vi "Test Parsing Simple Example Whlie Loop Some Operations 2.vi"() -> ()   [LabVIEW 2014]
panel:
  out "Transcripted code":string
  out "SubVI C calls":string[](array[string])
  out "error out 2":errorcluster
  out "WhileLoop C calls":string[](array[string])
  out "element translation order":string[](array[string])
  in  "vi path":path=path "C:/Users/lubo/Documents/LabView/LabVIEW-Universal-Transcriptor/Test/Examples For Parsing/Example While Loop Some Operations 2.vi"
  # "Everything is for noqw stored inside string list, so it means that all callected WhileLoops, SubVIs transcripted C code are store separately and after parsing there is generating them to output, but they are interleaved instead recursive nested, so this is what needs to repair next."
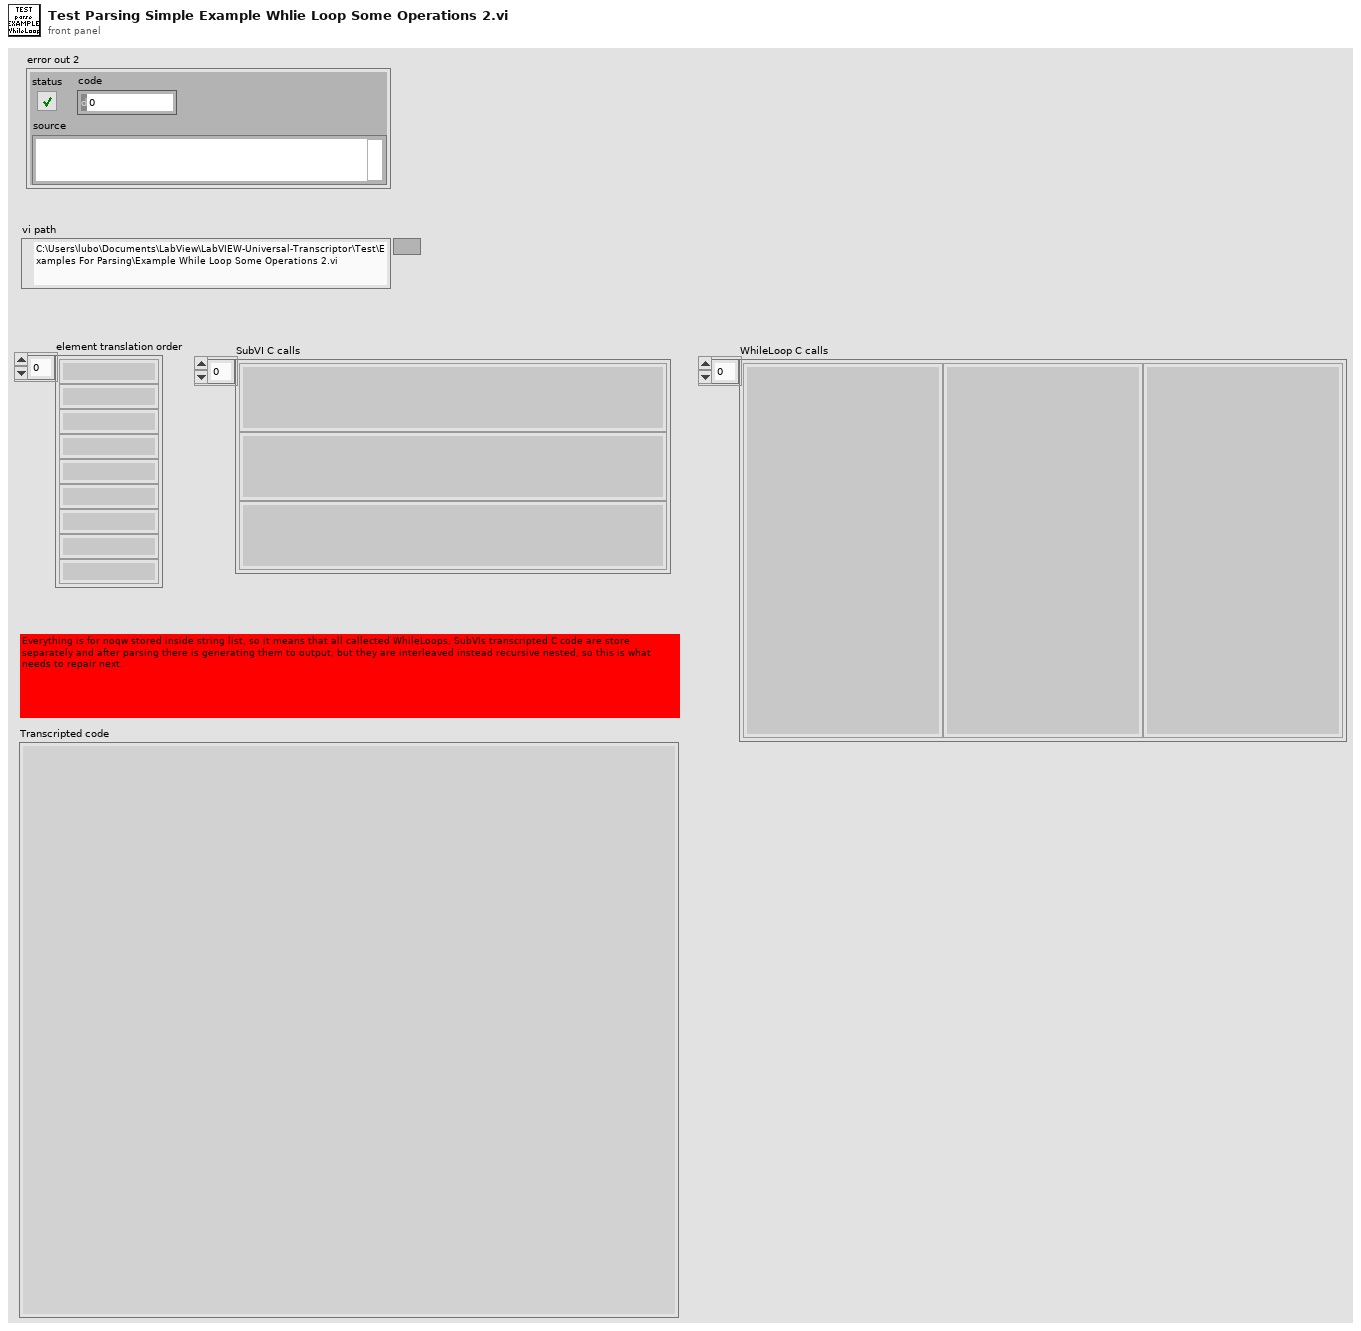
[diagram p1: front panel]
types:
  T1 = cluster{"terminals datatypes":string[][], "terminal\nconnected?":bool[], "terminal captions":string[], "term. count":i32, "terminal\nIsSource?":bool[], "SubVI name":string, "connected\nwires refs.":refnum<vi>[], "coerced\ndot?":bool[], "terminals[]":refnum<vi>[]}
  T2 = cluster{"terminals datatypes":string[][], "terminal\nconnected?":bool[], "terminal captions":string[], "term. count":i32, "terminal\nIsSource?":bool[], "SubVI name":string, "connected\nwires refs.":refnum<vi>[], "coerced dot?":bool[], "terminals[]":refnum<vi>[]}
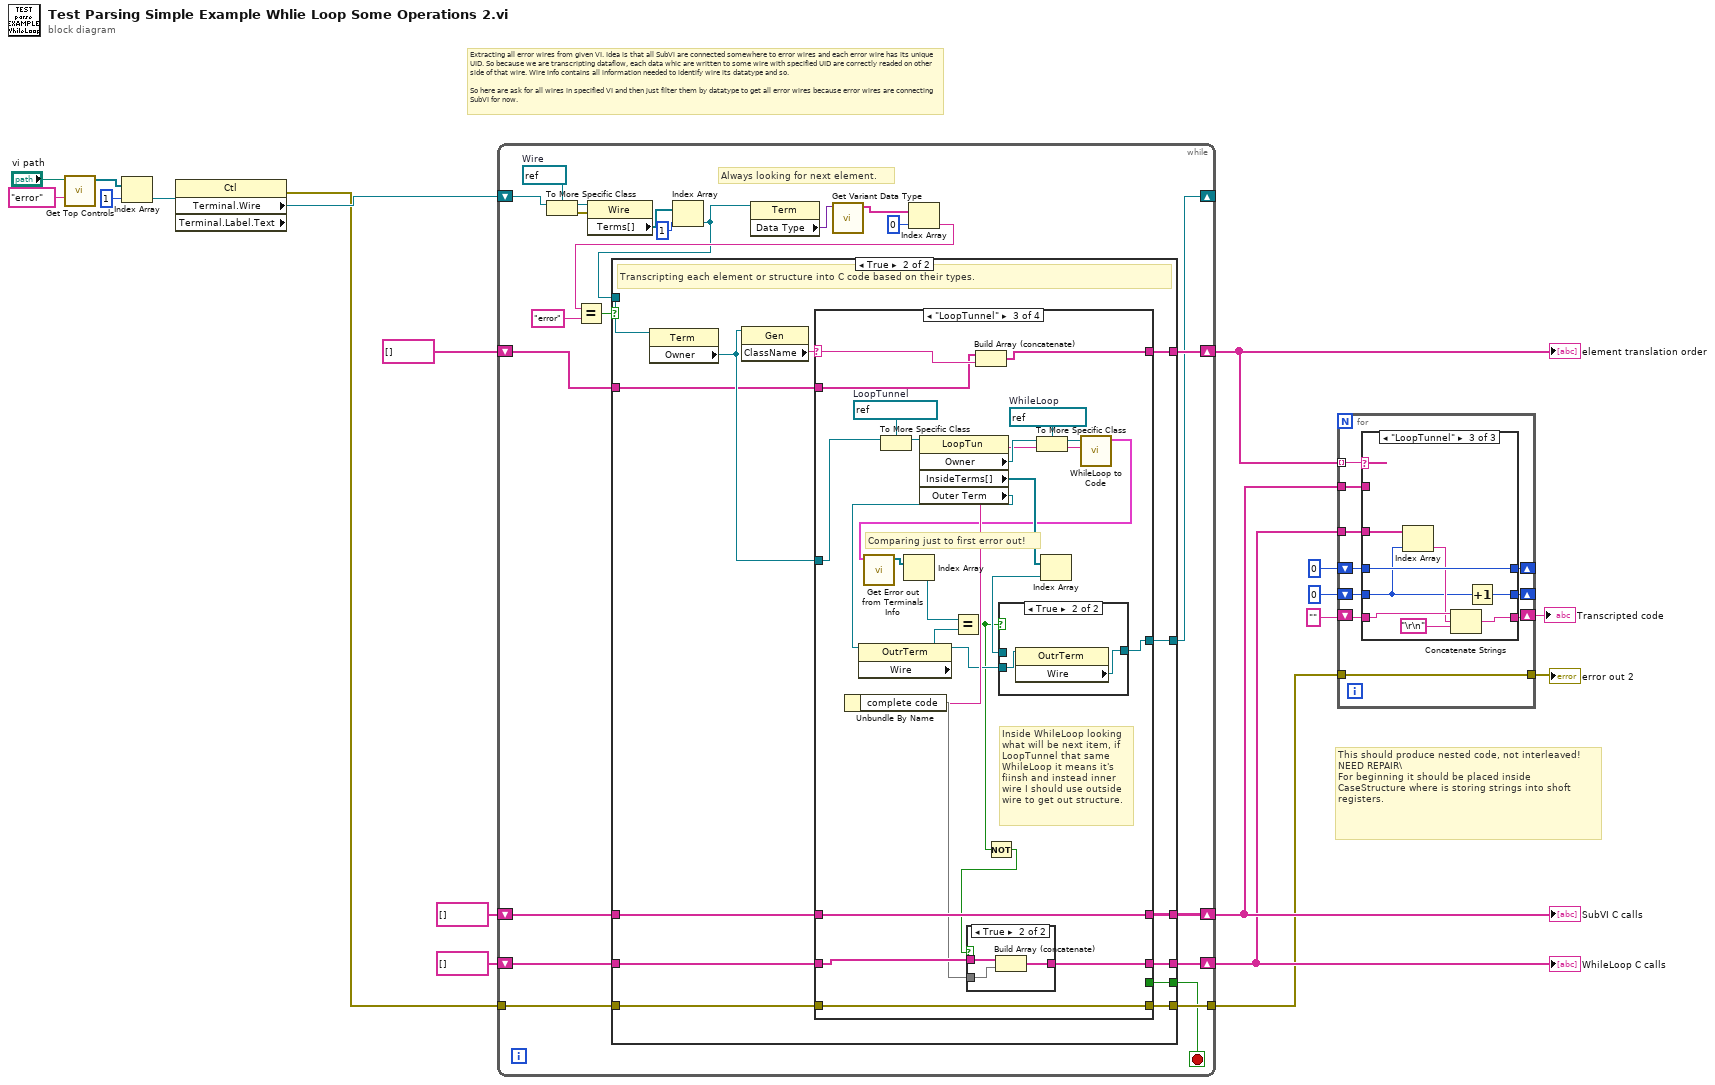
[diagram p0: block diagram]
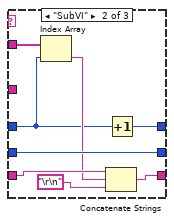
[diagram p3: hidden frame]
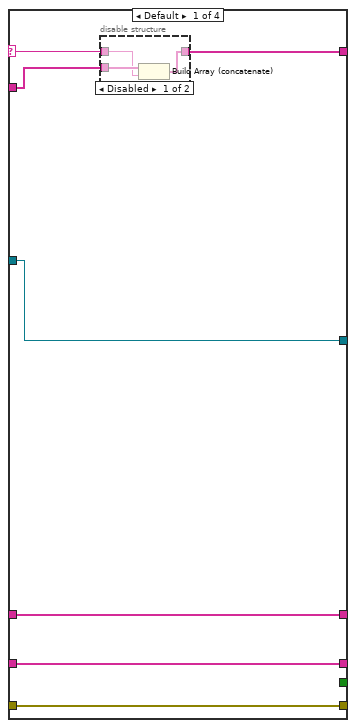
[diagram p5: hidden frame]
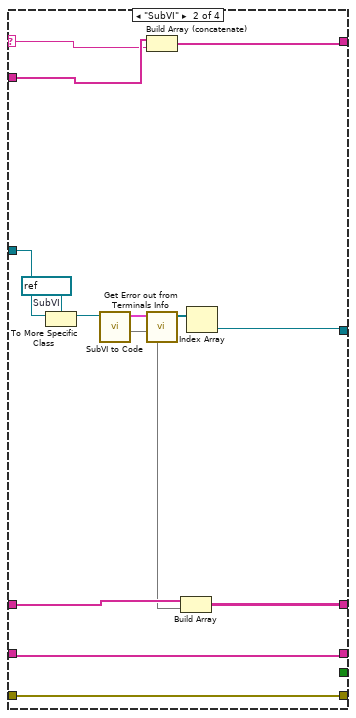
[diagram p7: hidden frame]
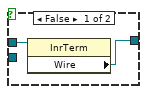
[diagram p9: hidden frame]
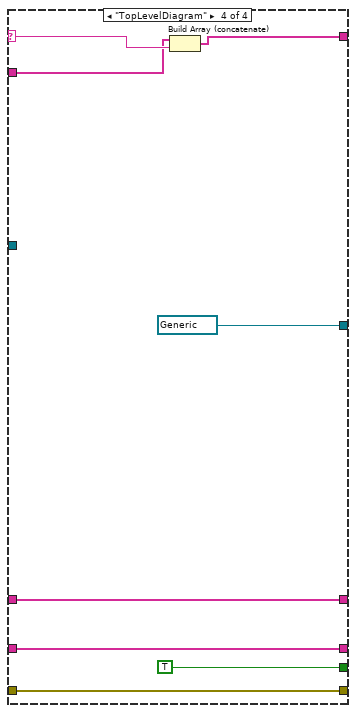
[diagram p10: hidden frame]
diagram:
  # "This should produce nested code, not interleaved!\nNEED REPAIR\\\nFor beginning it should be placed inside CaseStructure where is storing strings into shoft registers."
  # "Extracting all error wires from given VI. Idea is that all SubVi are connected somewhere to error wires and each error wire has its unique UID. So because we are transcripting dataflow, each data whic are written to some wire with specified UID are correctly readed on other side of that wire. Wire info contains all information needed to identify wire its datatype and so.\n\nSo here are ask for all wires in specified VI and then just filter them by datatype to get all error wires because error wires are connecting SubVI for now."
  n1 = call "Get Top Controls.vi"("DataType"="error", "vi path"="vi path") -> ("Controls Referencies Array"=w16:refnum<vi>[])  [unwired: 8 in, 1 out]
  n2 = Index Array(array=w16, index=1) -> (element=w15:refnum<vi>)
  n3 = property class="Ctl" props=["Terminal", "Wire", "Terminal", "Label", "Text"](reference=w15) -> (error out=w12:errorcluster, "Terminal.Wire"=w14:refnum<vi>)  [unwired: 1 in, 2 out]
  n4 = while {
    shift-right: [w31] -> w8
    shift-left: string[] [] -> [w30]
    shift-right: [w27] -> w7
    shift-left: string[] [] -> [w28]
    shift-right: [w26] -> w9
    shift-left: string[] [] -> [w25]
    tunnel: [w23] -> w2
    tunnel: w12 -> [w22]
    shift-right: [w21] -> _
    shift-left: w14 -> [w24]
    stop <- w20 stop-if-true
    w42 = refnum<vi> refnum  # Wire
    # "Always looking for next element."
    n5 = To More Specific Class(target class=w42, reference=w24) -> (specific class reference=w33:refnum<vi>, error out=w41:errorcluster)  [unwired: 1 in]
    n6 = property class="Wire"(reference=w33, error in=w41) -> ("Terms[]"=w40:refnum<vi>[])  [unwired: 2 out]
    n7 = Index Array(array=w40, index=1) -> (element=w29:refnum<vi>)
    n8 = property class="Term"(reference=w29) -> ("Data Type"=w39:variant)  [unwired: 1 in, 2 out]
    n9 = call "Get Variant Data Type.vi"("Variant in"=w39) -> ("Data Types[]"=w38:string[])  [unwired: 9 in, 1 out]
    n10 = Index Array(array=w38, index=0) -> (element=w36:string)
    n11 = Equal?(x=w36, y="error") -> (x = y?=w32:bool)
    n12 = case shown="True" w32 {
      tunnel: [w47 w59] -> w31
      tunnel: w30 -> [w47 w58]
      tunnel: w29 -> [w43 w57]
      tunnel: w28 -> [w46 w55]
      tunnel: [w46 w54] -> w27
      tunnel: [w45 w53] -> w26
      tunnel: w25 -> [w45 w52]
      tunnel: [w44 w51] -> w23
      tunnel: w22 -> [w44 w50]
      tunnel: [w43 w49] -> w21
      tunnel: [_ w48] -> w20
      frame False {
      }
      frame True {
        # "Transcripting each element or structure into C code based on their types."
        n13 = property class="Term"(reference=w57) -> ("Owner"=w60:refnum<vi>)  [unwired: 1 in, 2 out]
        n14 = property class="Gen"(reference=w60) -> ("ClassName"=w56:string)  [unwired: 1 in, 2 out]
        n15 = case shown="\"LoopTunnel\"" w56 {
          selector: w56 -> [w64 w79 w106 w125]
          tunnel: w60 -> [w61 w84 w103 _]
          tunnel: [w67 w82 w110 w127] -> w59
          tunnel: w58 -> [w67 w83 w110 w127]
          tunnel: w55 -> [w66 w81 w108 w121]
          tunnel: [w66 w81 w109 w121] -> w54
          tunnel: [w63 w78 w107 w126] -> w53
          tunnel: w52 -> [w65 w80 w105 w124]
          tunnel: [w62 w77 w100 w123] -> w51
          tunnel: w50 -> [w62 w77 w100 w123]
          tunnel: [w61 w72 w94 refnum<vi> refnum ("Owner")] -> w49
          tunnel: [_ _ _ TRUE] -> w48
          frame Default {
            n16 = disable-structure shown="Disabled" {
              disable-tunnel: w65 -> [w70 w71]
              disable-tunnel: w64 -> [w69 _]
              disable-tunnel: [w68 w71] -> w63
              frame Disabled {
                n17 = Build Array (concatenate)(w70, w69) -> (w68:string[])
              }
              frame Enabled {
              }
            }
          }
          frame "SubVI" {
            w85 = refnum<vi> refnum  # SubVI
            n18 = To More Specific Class(target class=w85, reference=w84) -> (specific class reference=w76:refnum<vi>)  [unwired: 1 in, 1 out]
            n19 = call "SubVI to Code.vi"("reference"=w76) -> (1:w75, "SubVI terminals info"=w73:T1)  [unwired: 8 in, 1 out]
            n20 = Build Array (concatenate)(w80, w79) -> (w78:string[])
            n21 = call "Get Error out from Terminals Info.vi"("terminals info"=w73) -> ("error out terminals"=w74:refnum<vi>[])  [unwired: 9 in, 1 out]
            n22 = Build Array(w83, w75) -> (w82:string[][])
            n23 = Index Array(array=w74) -> (element=w72:refnum<vi>)  [unwired: 1 in]
          }
          frame "LoopTunnel" {
            w104 = refnum<vi> refnum  # LoopTunnel
            w111 = refnum<vi> refnum  # WhileLoop
            # "Comparing just to first error out!"
            # "Inside WhileLoop looking what will be next item, if LoopTunnel that same WhileLoop it means it's fiinsh and instead inner wire I should use outside wire to get out structure."
            n24 = To More Specific Class(target class=w104, reference=w103) -> (specific class reference=w102:refnum<vi>)  [unwired: 1 in, 1 out]
            n25 = property class="LoopTun"(reference=w102) -> ("Owner"=w101:refnum<vi>, "InsideTerms[]"=w96:refnum<vi>[], "Outer Term"=w91:refnum<vi>)  [unwired: 1 in, 2 out]
            n26 = property class="OutrTerm"(reference=w91) -> (reference out=w88:refnum<vi>, "Wire"=w89:refnum<vi>)  [unwired: 1 in, 1 out]
            n27 = Build Array (concatenate)(w105, w106) -> (w107:string[])
            n28 = To More Specific Class(target class=w111, reference=w101) -> (specific class reference=w97:refnum<vi>)  [unwired: 1 in, 1 out]
            n29 = Index Array(array=w96) -> (element=w95:refnum<vi>)  [unwired: 1 in]
            n30 = call "WhileLoop to Code.vi"("WhileLoop ref"=w97) -> ("C code"=w98:string, "terminals info"=w93:T2)  [unwired: 8 in, 1 out]
            n31 = Unbundle By Name(w98) -> ("complete code"=w99)
            n32 = call "Get Error out from Terminals Info.vi"("terminals info"=w93) -> ("error out terminals"=w92:refnum<vi>[])  [unwired: 9 in, 1 out]
            n33 = Index Array(array=w92) -> (element=w90:refnum<vi>)  [unwired: 1 in]
            n34 = Equal?(x=w90, y=w89) -> (x = y?=w86:bool)
            n35 = Not(x=w86) -> (.not. x?=w87:bool)
            n36 = case shown="True" w87 {
              tunnel: [w112 w115] -> w109
              tunnel: w108 -> [w112 w114]
              tunnel: w99 -> [_ w113]
              frame False {
              }
              frame True {
                n37 = Build Array (concatenate)(w114, w113) -> (w115:string[])
              }
            }
            n38 = case shown="True" w86 {
              tunnel: w95 -> [w117 _]
              tunnel: [w116 w118] -> w94
              tunnel: w88 -> [_ w119]
              frame False {
                n39 = property class="InrTerm"(reference=w117) -> ("Wire"=w116:refnum<vi>)  [unwired: 1 in, 2 out]
              }
              frame True {
                n40 = property class="OutrTerm"(reference=w119) -> ("Wire"=w118:refnum<vi>)  [unwired: 1 in, 2 out]
              }
            }
          }
          frame "TopLevelDiagram" {
            n41 = Build Array (concatenate)(w124, w125) -> (w126:string[])
          }
        }
      }
    }
  }
  "element translation order" <- w9
  "WhileLoop C calls" <- w7
  "SubVI C calls" <- w8
  n42 = for {
    tunnel: w9 -> [w137] mode=indexing
    tunnel: w8 -> [w136]
    tunnel: w7 -> [w135]
    shift-right: [w132] -> _
    shift-left: 0 -> [w131]
    shift-right: [w133] -> _
    shift-left: 0 -> [w134]
    shift-right: [w129] -> w3
    shift-left: "" -> [w130]
    tunnel: [w128] -> w1
    tunnel: w2 -> [w128]
    n43 = case shown="\"LoopTunnel\"" w137 {
      tunnel: w136 -> [_ w146 _]
      tunnel: w135 -> [_ _ w154]
      tunnel: w134 -> [w140 w148 w150]
      tunnel: [w140 w148 w155] -> w133
      tunnel: [w139 w147 w156] -> w132
      tunnel: w131 -> [w139 w141 w156]
      tunnel: w130 -> [w138 w144 w152]
      tunnel: [w138 w145 w153] -> w129
      frame Default {
      }
      frame "SubVI" {
        n44 = Index Array(array=w146, index=w141) -> (element=w143:string)
        n45 = Concatenate Strings(w144, w143, "\r\n") -> (w145:string)
        n46 = Increment(x=w141) -> (x+1=w147:i32)
      }
      frame "LoopTunnel" {
        n47 = Index Array(array=w154, index=w150) -> (element=w151:string)
        n48 = Concatenate Strings(w152, w151, "\r\n") -> (w153:string)
        n49 = Increment(x=w150) -> (x+1=w155:i32)
      }
    }
  }
  "error out 2" <- w1
  "Transcripted code" <- w3
